vi "CRYCalc Voltage on DUT.vi"(9 "VL":dbl, 10 "Rn":dbl, 11 "Ro":dbl) -> (3 "Vo":dbl)   [LabVIEW 2013]
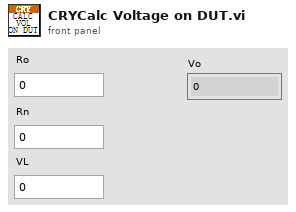
[diagram p1: front panel]
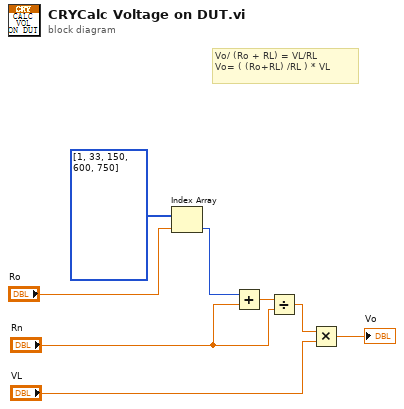
[diagram p0: block diagram]
diagram:
  # "Vo/ (Ro + RL) = VL/RL\nVo= ( (Ro+RL) /RL ) * VL"
  n1 = Index Array(array=i32[] [1, 33, 150, 600, 750], index="Ro") -> (element=w1:i32)
  n2 = Add(x=w1, y="Rn") -> (x+y=w7:dbl)
  n3 = Divide(x=w7, y="Rn") -> (x/y=w6:dbl)
  n4 = Multiply(x=w6, y="VL") -> (x*y=→"Vo":dbl)
